vi "Excel Insert Header.vi"(7 "시트명":string="교정결과", 8 "error in":errorcluster caption="에러 입력(에러 없음)", 11 "report in":refnum<class "NI_report.lvclass">) -> (0 "error out":errorcluster, 3 "report out":refnum<class "NI_report.lvclass">, 4 "삭제에러":bool)   [LabVIEW 2020]
uses:
  <vilib>/Utility/NIReport.llb/NI_report.lvclass
  Controls/Cmd_Excel Insert Header.ctl
  <vilib>/Utility/error.llb/DialogType.ctl
  <vilib>/addons/_office/excel.llb/Excel Get Data ([str]).vi
  Variables/Global_Cal Info.vi
  <vilib>/Utility/error.llb/Error Cluster From Error Code.vi
  <vilib>/ErrorRing/Error Ring.xnode
  <vilib>/Utility/NIReport.llb/Excel/NI_Excel.lvclass
  <vilib>/addons/_office/NI_ReportGenerationToolkit.lvlib
panel:
  out "Header Lower":i32
  out "Header Upper":i32
  out "배열":string[][][](array[string])
  out "원소":string
  out "원소의 인덱스":i32
  out "Line":i32
  out "B_Tag Upper":i32
  out "B_Tag Lower":i32
  out "Header Column":i32
  out "?":T1
  out "Header Column":i32[](array[numeric])
  out "Header Row Count":i32[](array[numeric])
  out "Header Row":i32[](array[numeric])
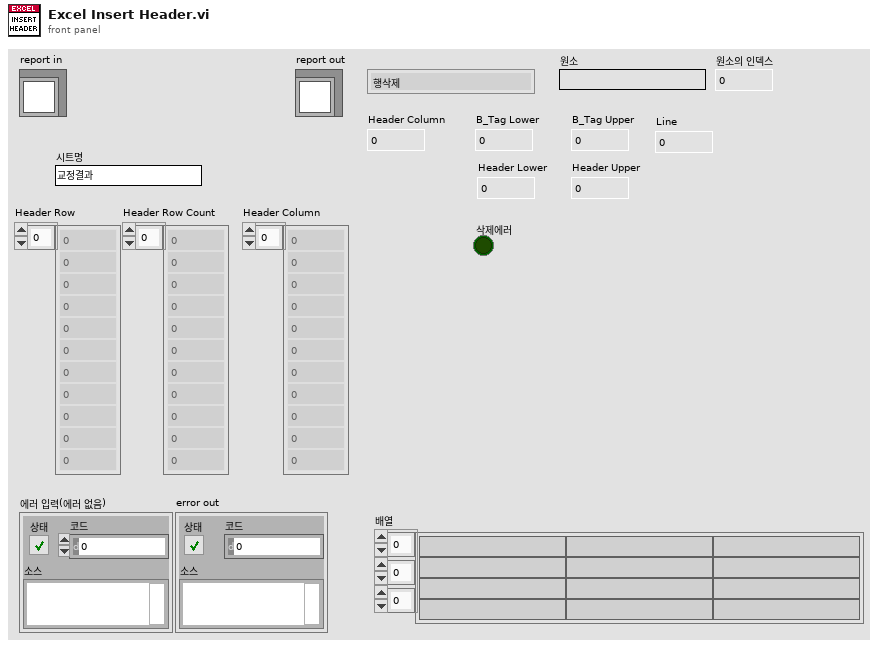
[diagram p1: front panel]
types:
  T1 = typedef "Cmd_Excel Insert Header.ctl" = enum16{"행삭제", "페이지 삭제", "B_Tag 읽기", "Header 읽기", "행 삽입", "Header 삽입", "Header 넘버링", "B_Tag 삽입", "오류 검사", "종료", "Error"}
  T2 = cluster{"position (excel)":cluster{"row":i32, "column":i32}, "name (excel)":string, "bookmark (word)":string}
  T3 = typedef "Clst_Cal Info Global.ctl" = cluster{"등록번호":string, "의뢰기관":string, "기기명":string, "제작회사":string, "형식":string, "기기번호":string, "소분류코드":string, "세부분류코드":string, "교정주기":string, "접수번호":string, "교정일자":string, "교정절차서 1":string, "교정절차서 2":string, "교정절차서 3":string, "접수확인자":string, "인증교정자":string, "기술책임자":string, "KOLAS 유무":string, "진행상태":string, "의뢰기관코드":string, "입고형태":string, "영문성적서?":bool, "합불판정?":bool, "부록?":bool, "절차서번호 1":string, "절차서번호 2":string, "절차서번호 3":string, "교정방식":string, "부서명":string}
  T4 = typedef "DialogType.ctl" = u16
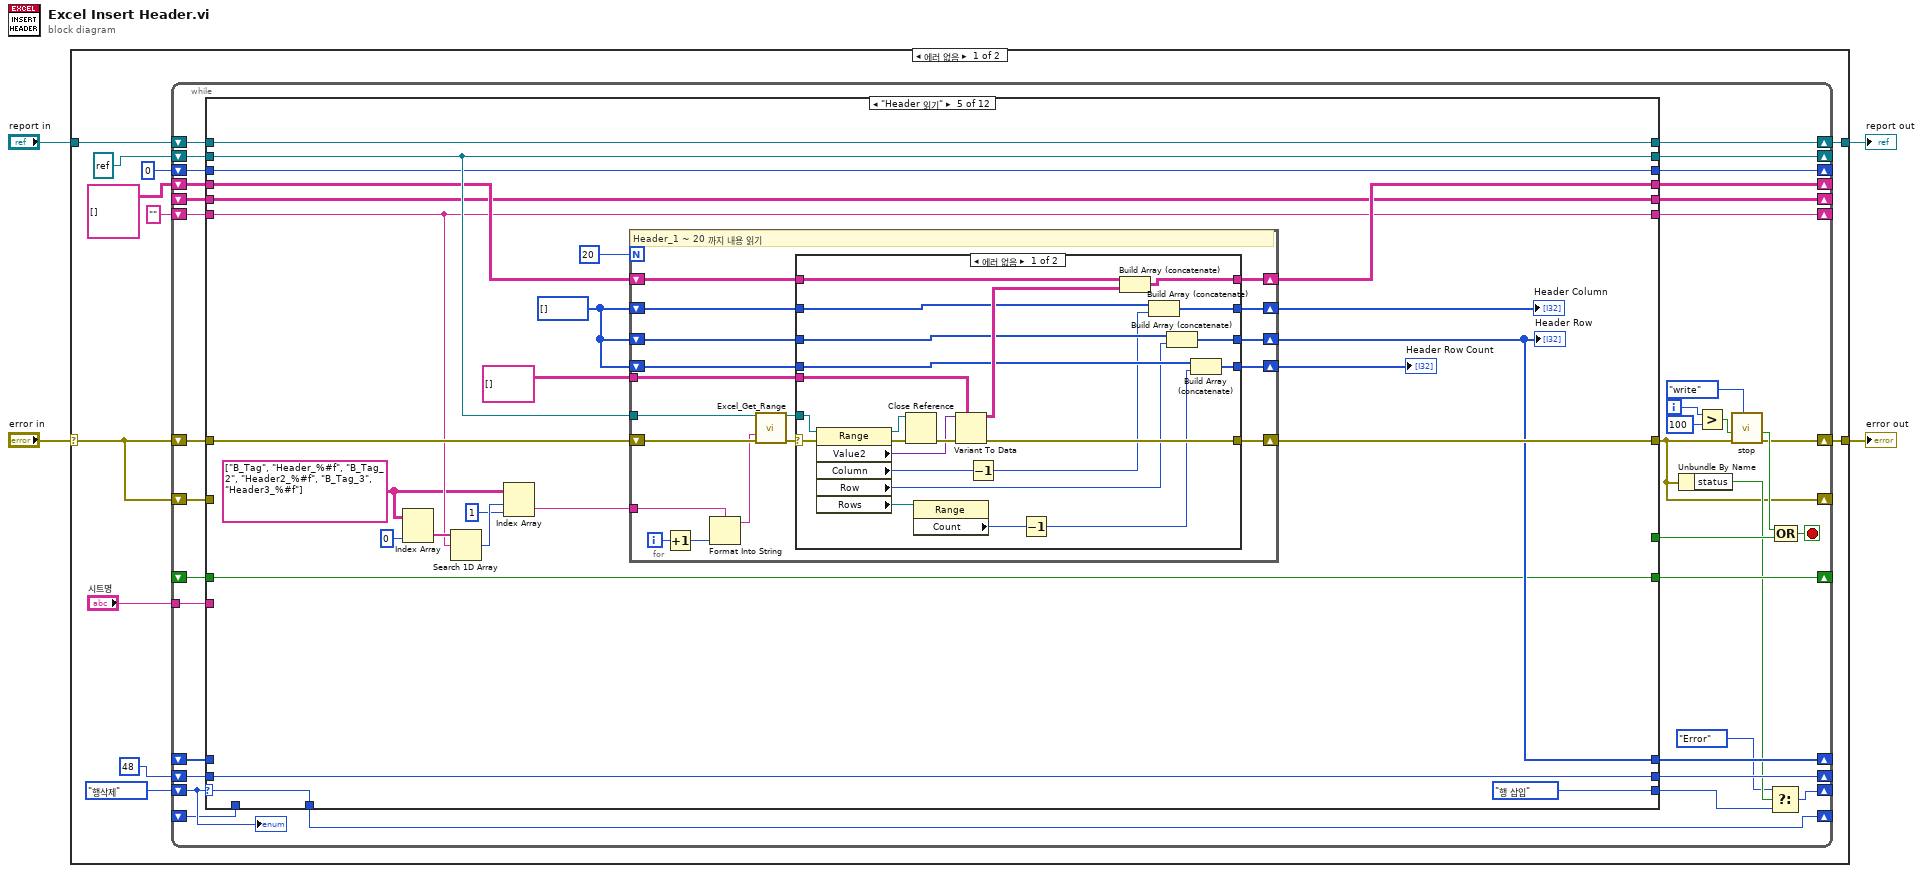
[diagram p0: block diagram]
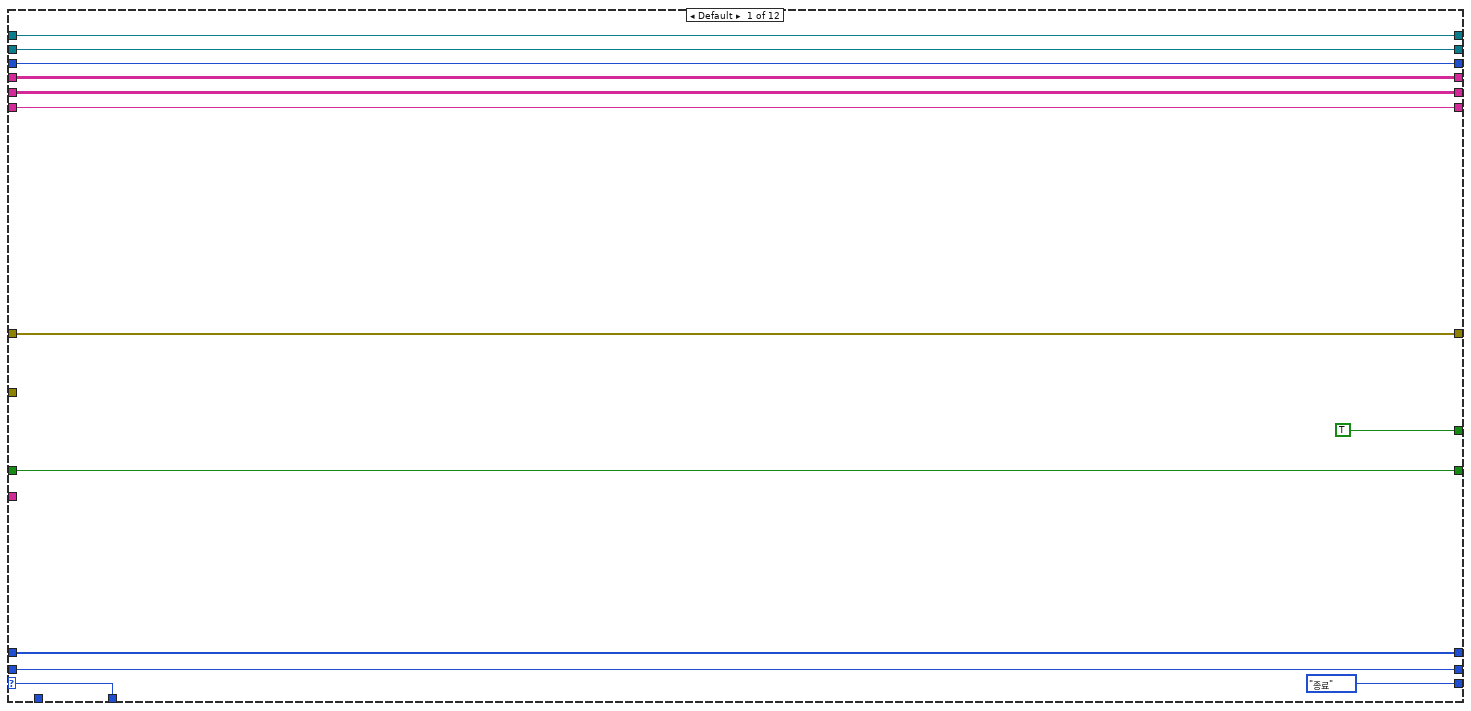
[diagram p2: hidden frame]
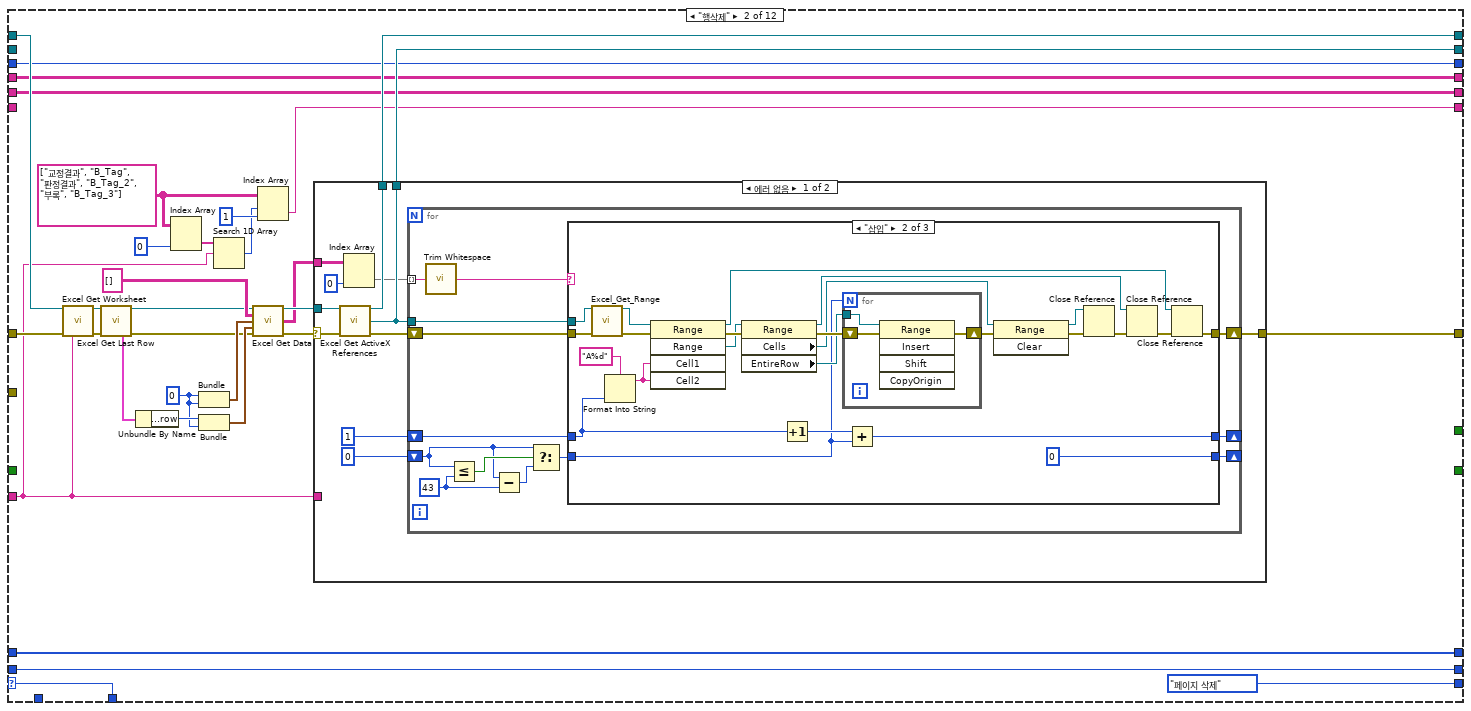
[diagram p3: hidden frame]
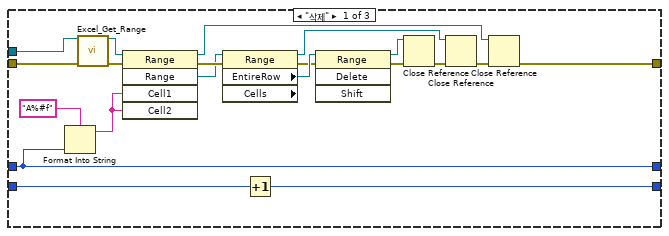
[diagram p4: hidden frame]
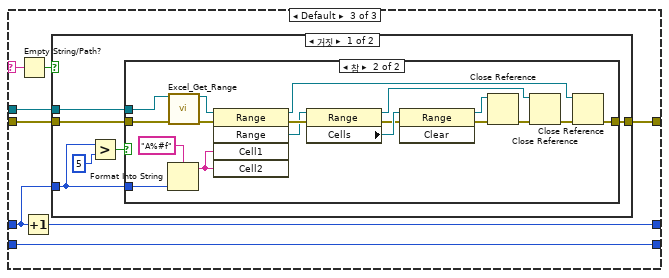
[diagram p5: hidden frame]
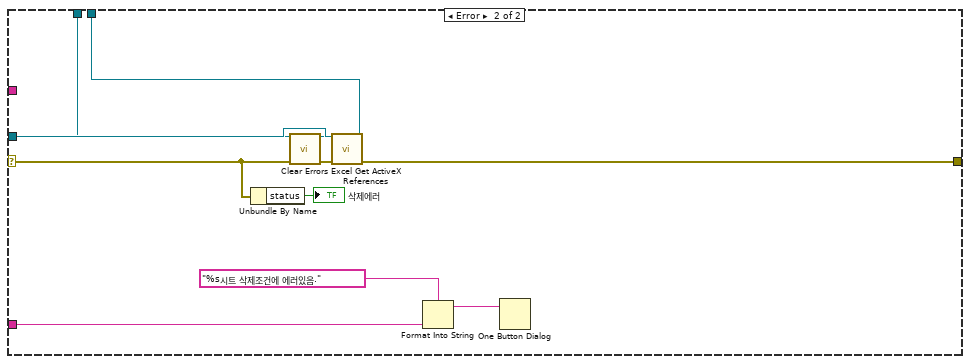
[diagram p8: hidden frame]
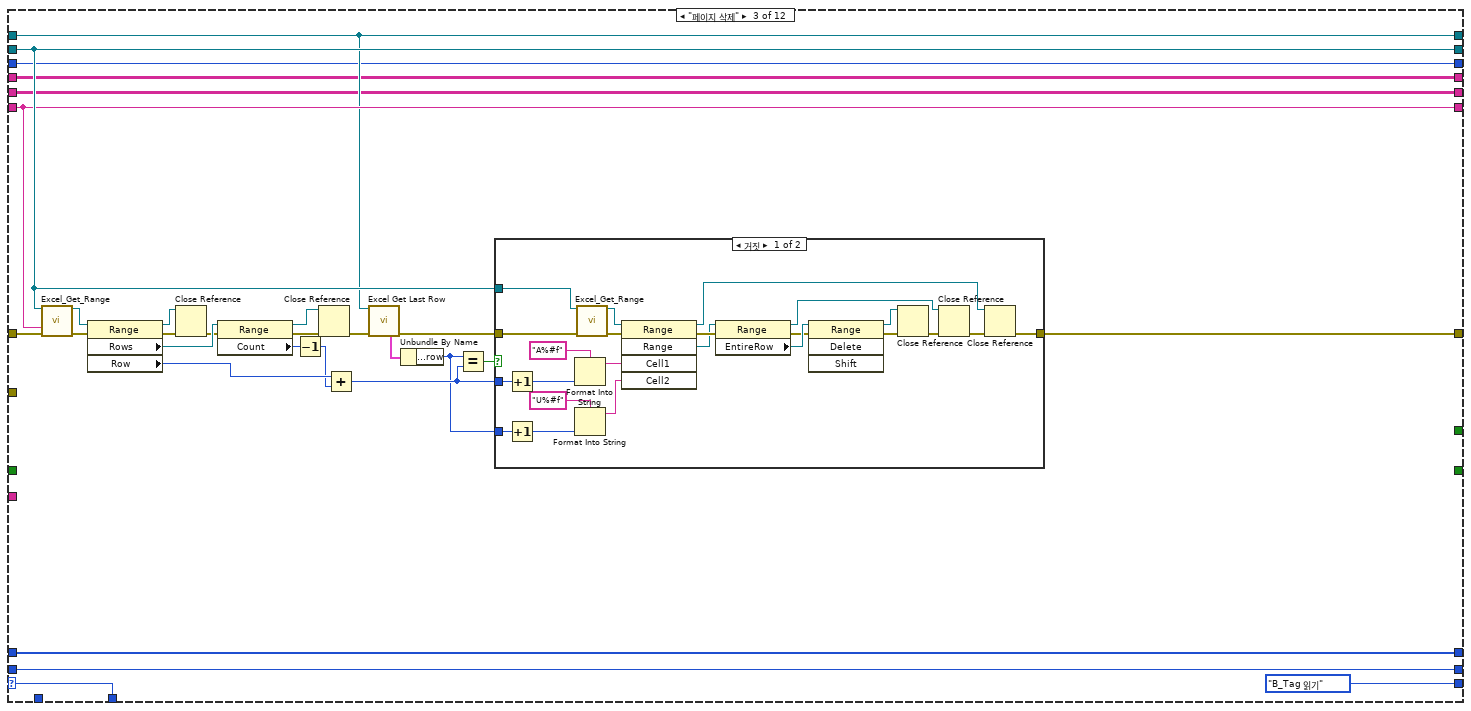
[diagram p9: hidden frame]
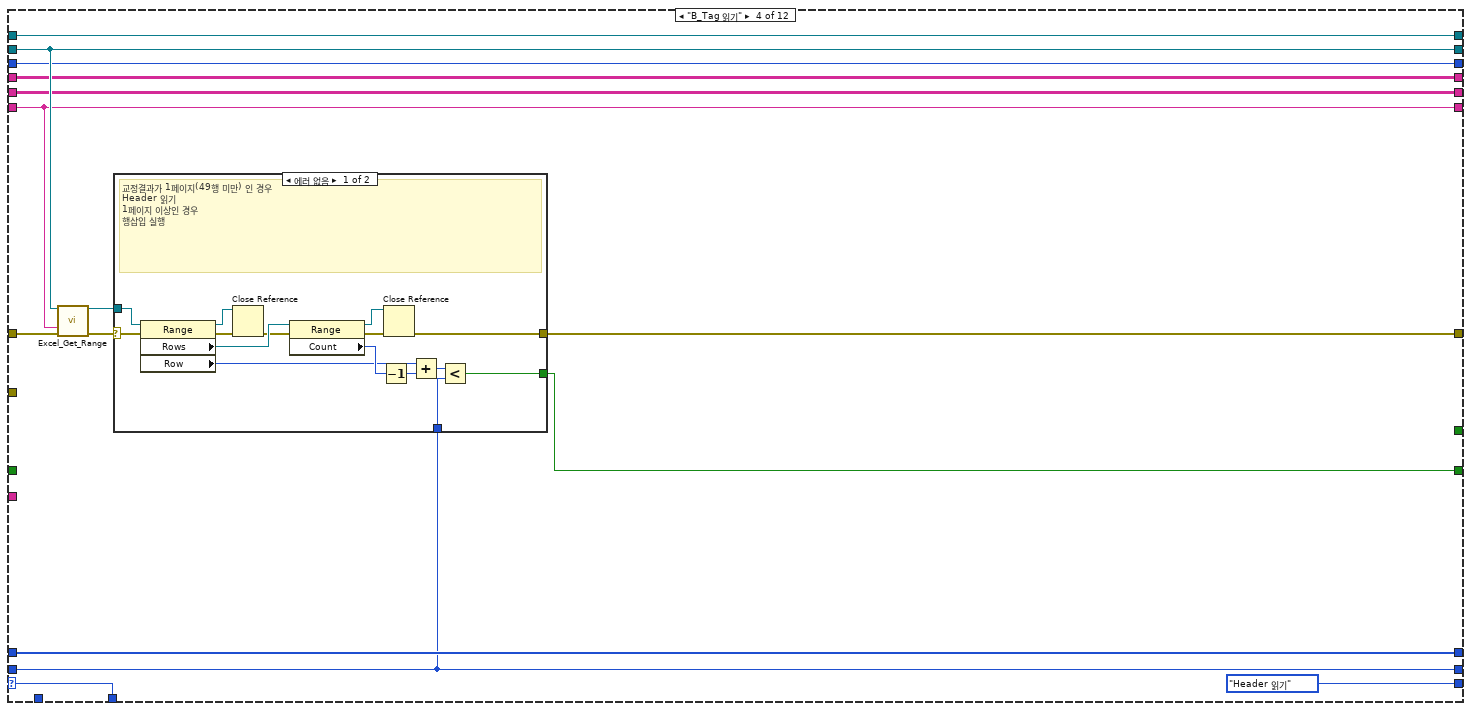
[diagram p11: hidden frame]
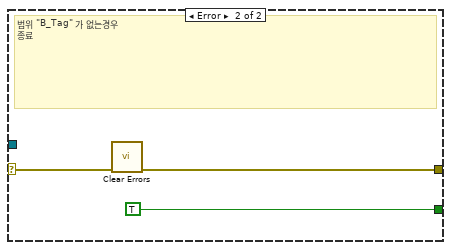
[diagram p12: hidden frame]
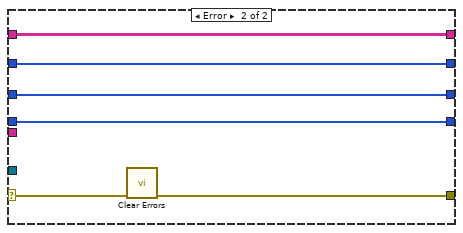
[diagram p13: hidden frame]
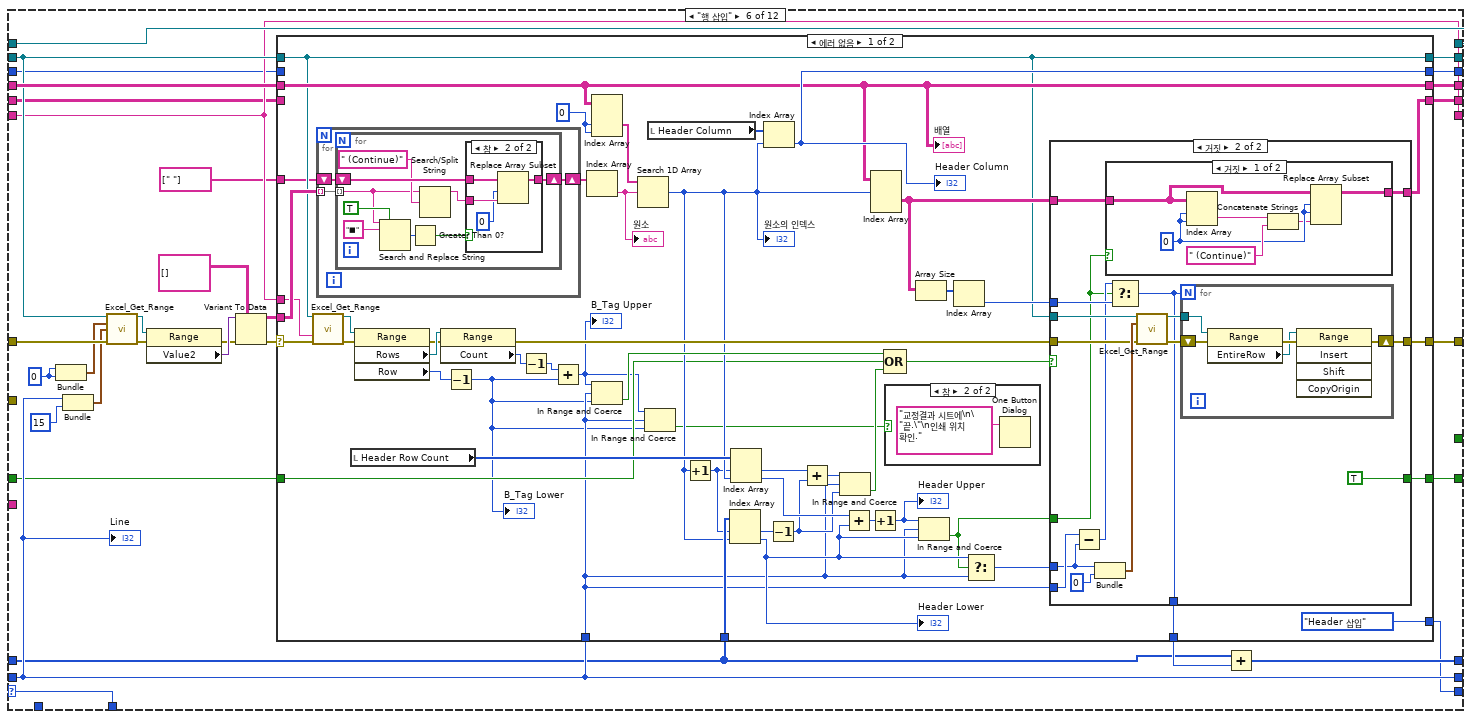
[diagram p14: hidden frame]
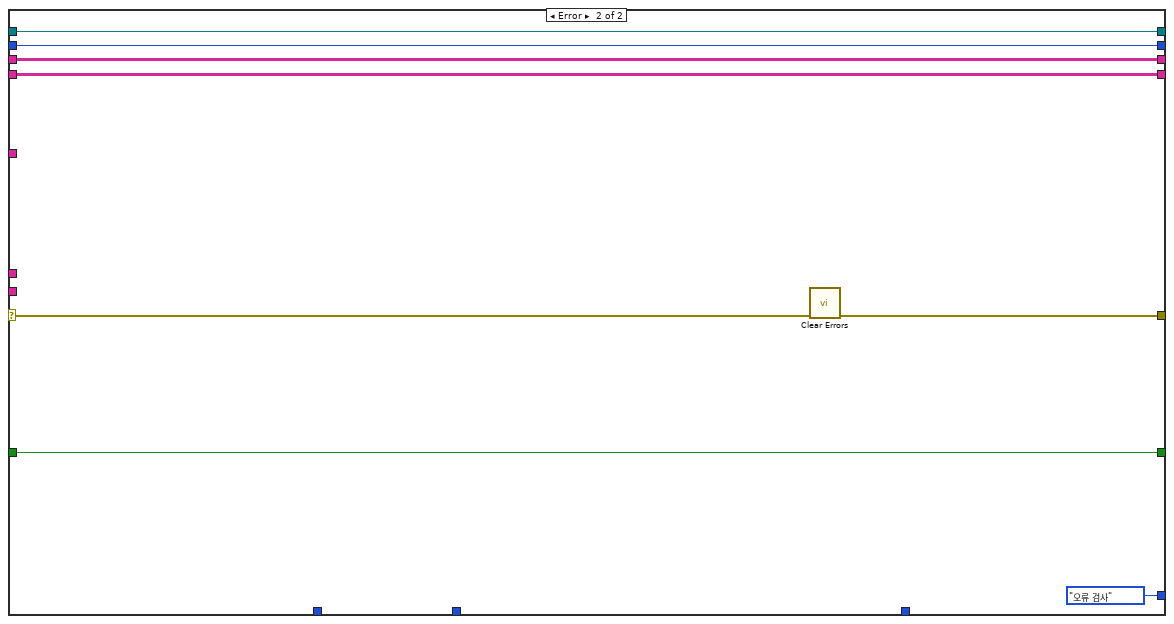
[diagram p19: hidden frame]
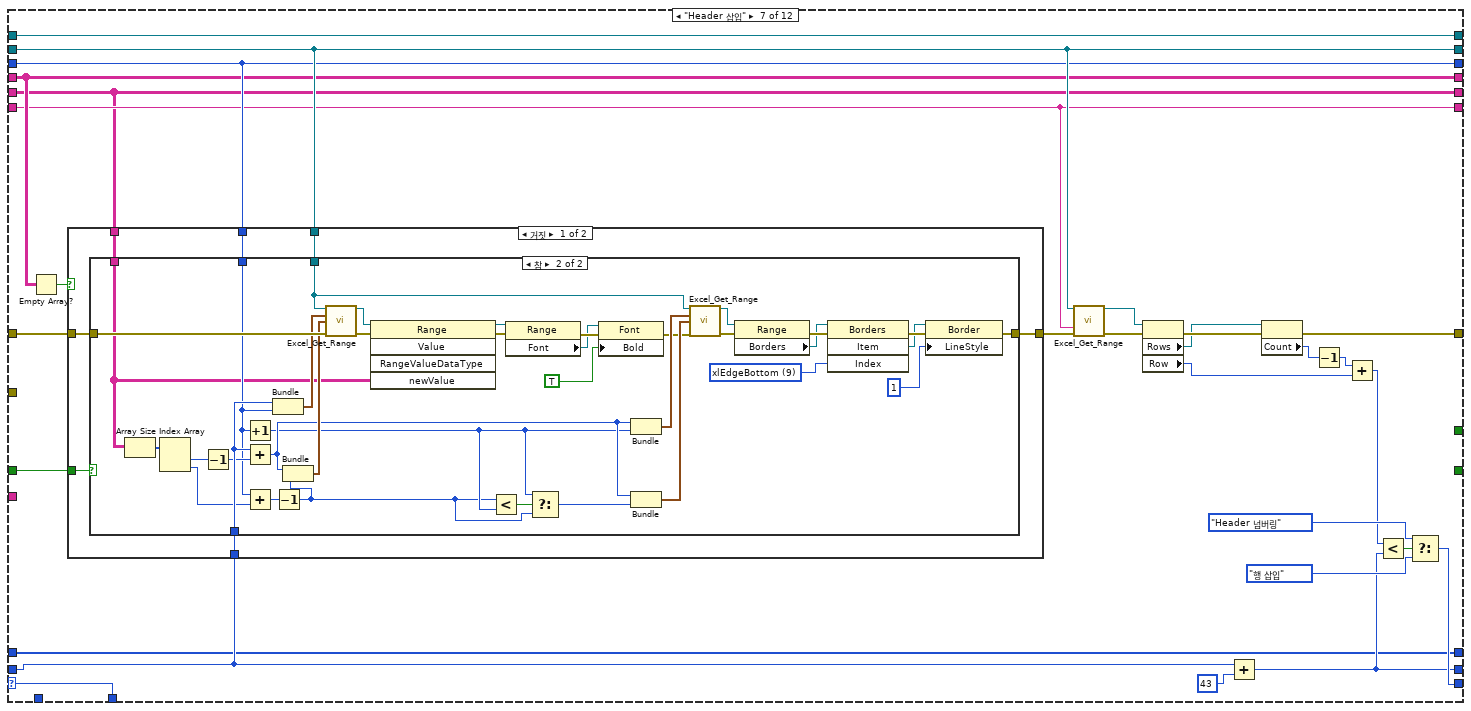
[diagram p20: hidden frame]
diagram:
  n1 = case shown="에러 없음" "error in" {
    selector: "error in" -> [w5 w784]
    tunnel: [w15 w784] -> w2
    tunnel: [w14 w783] -> w3
    tunnel: "report in" -> [w9 w783]
    frame No Error {
      n2 = while {
        shift-right: [w38] -> _
        shift-left: 48 -> [w29]
        shift-right: [w35] -> w15
        shift-left: w5 -> [w52]
        shift-right: [w22] -> _
        shift-left: Cmd_Excel_Insert_Header."행삭제" -> [w30]
        shift-right: [w51] -> w14
        shift-left: w9 -> [w50]
        shift-right: [w49] -> _
        shift-left: refnum<k7> refnum ("Excel._Worksheet") -> [w48]
        shift-right: [w47] -> _
        shift-left: string[][][] [] -> [w46]
        shift-right: [w37] -> _
        shift-left: 0 ("Column") -> [w36]
        shift-right: [w34] -> _
        shift-left: _ -> [w31]
        shift-right: [w32] -> _
        shift-left: _ -> [w33]
        shift-right: [w27] -> _
        shift-left: _ -> [w28]
        shift-right: [w25] -> _
        shift-left: "" -> [w26]
        tunnel: "시트명" -> [w24]
        shift-right: [w20] -> _
        shift-left: w5 -> [w19]
        shift-right: [w16] -> _
        shift-left: _ -> [w17]
        i -> [w42]
        stop <- w45 stop-if-true
        n3 = case shown="\"Header 읽기\"" w30 {
          selector: w30 -> [w53 w67 w213 w266 w299 w371 w508 w581 w663 w714 w748 w760]
          tunnel: [w55 w81 w223 w273 w317 w384 w517 w591 w702 w721 w753 w770] -> w38
          tunnel: w52 -> [w59 w86 w240 w276 w322 w401 w530 w600 w707 w727 w755 _]
          tunnel: [Cmd_Excel_Insert_Header."종료" Cmd_Excel_Insert_Header."페이지 삭제" Cmd_Excel_Insert_Header."B_Tag 읽기" Cmd_Excel_Insert_Header."Header 읽기" Cmd_Excel_Insert_Header."행 삽입" w378 w533 Cmd_Excel_Insert_Header."B_Tag 삽입" Cmd_Excel_Insert_Header."오류 검사" Cmd_Excel_Insert_Header."종료" Cmd_Excel_Insert_Header."종료" Cmd_Excel_Insert_Header."종료"] -> w18
          tunnel: [w65 w88 w222 w277 w320 w402 w532 w585 w706 w716 w759 w775] -> w51
          tunnel: w50 -> [w65 w84 w222 w277 w320 w402 w532 w599 w706 w725 w759 w775]
          tunnel: [w64 w87 w237 w275 w321 w374 w528 w596 w691 w724 w758 w774] -> w49
          tunnel: w48 -> [w64 _ w237 w275 w321 w386 w528 w596 w691 w724 w758 w774]
          tunnel: [w59 w80 w241 w278 w319 w392 w519 w586 w704 w726 w755 w764] -> w20
          tunnel: [w62 w75 w215 w268 w318 w379 w514 w592 w703 w722 w754 w771] -> w47
          tunnel: w46 -> [w62 w75 w215 w268 w311 w393 w514 w592 w703 w722 w754 w771]
          tunnel: [TRUE _ _ _ _ _ _ _ _ _ TRUE TRUE] -> w44
          tunnel: [w63 w76 w216 w269 w308 w388 w527 w587 w700 w718 w750 w767] -> w37
          tunnel: w36 -> [w63 w76 w216 w269 w308 w375 w527 w587 w700 w718 w750 w767]
          tunnel: [w58 _ _ w271 w307 w389 _ _ _ _ _ _] -> w34
          tunnel: w33 -> [w61 w74 w214 w267 w309 w373 w509 w588 w664 w717 w749 w766]
          tunnel: [w61 w74 w214 w267 w309 w387 w509 w588 w664 w717 w749 w766] -> w32
          tunnel: w31 -> [w58 _ _ _ w307 w377 w511 _ _ _ _ _]
          tunnel: w29 -> [w55 w81 w223 w273 w317 w384 w526 w591 w702 w721 w753 w770]
          tunnel: w28 -> [w56 w82 w239 w274 _ w381 w515 w590 w701 w720 w752 w769]
          tunnel: [w56 w82 w239 w274 w315 w382 w515 w590 w701 w720 w752 w769] -> w27
          tunnel: w26 -> [w60 _ w225 w270 w304 w376 w512 w589 w699 w719 w751 w768]
          tunnel: [w60 w68 w225 w270 w304 w376 w512 w589 w699 w719 w751 w768] -> w25
          tunnel: w24 -> [_ w66 _ _ _ _ _ _ _ w715 _ _]
          tunnel: w19 -> [_ _ _ _ _ _ _ _ _ _ _ _]
          tunnel: w17 -> [_ _ _ _ _ _ _ _ _ _ _ w761]
          tunnel: [w53 w67 w213 w266 w299 w371 w508 w581 w663 w714 w748 w760] -> w16
          frame Default {
          }
          frame "행삭제" {
            w71 = string[][] [["교정결과", "B_Tag"], ["판정결과", "B_Tag_2"], ["부록", "B_Tag_3"]]
            w78 = 0
            n4 = call <vilib>:"Excel Get Worksheet.vi"("report in"=w84, "error in (no error)"=w86, "name (\"\")"=w66) -> ("report out"=w83:refnum<class "NI_report.lvclass">, "error out"=w85:errorcluster)  [unwired: 11 in]
            n5 = call <vilib>:"Excel Get Last Row.vi"("report in"=w83, "error in (no error)"=w85) -> ("report out"=w91:refnum<class "NI_report.lvclass">, "MS Office parameters out"=w90:T2, "error out"=w92:errorcluster)  [unwired: 11 in]
            n6 = Unbundle By Name(w90) -> ("position (excel).row"=w95:i32)
            n7 = Index Array(array=w71, index (col)=0 ("비활성화된 인덱스 (열)")) -> (element=w72:string[])  [unwired: 1 in]
            n8 = Bundle(w78, w78) -> (w94:cluster{i32, i32})  [unwired: 1 in]
            n9 = Bundle("row"=w95, w78) -> (w96:cluster{"row":i32, i32})  [unwired: 1 in]
            n10 = Search 1D Array(1D array=w72, element=w66) -> (index of element=w69:i32)  [unwired: 1 in]
            n11 = call-poly <vilib>:"Excel Get Data.vi"("report in"=w91, "data type"=string[][] [], "start (-1, -1)"=w94, "end (-1, -1)"=w96, "error in (no error)"=w92) -> ("report out"=w97:refnum<class "NI_report.lvclass">, "data"=w89:string[][], "error out"=w79:errorcluster)  [unwired: 8 in]
            n12 = Index Array(array=w71, index (row)=w69, index (col)=1 ("비활성화된 인덱스 (열)")) -> (element=w68:string)
            n13 = case shown="에러 없음" w79 {
              selector: w79 -> [w101 w207]
              tunnel: w97 -> [w108 w212]
              tunnel: w89 -> [w100 _]
              tunnel: [w106 w211] -> w88
              tunnel: [w105 w210] -> w87
              tunnel: [w102 w209] -> w80
              tunnel: w66 -> [_ w205]
              frame No Error {
                n14 = call <vilib>:"Excel Get ActiveX References.vi"("report in"=w108, "error in (no error)"=w101) -> ("report out"=w106:refnum<class "NI_report.lvclass">, "Excel._Worksheet"=w105:refnum<k7>, "error out"=w107:errorcluster)  [unwired: 7 in, 4 out]
                n15 = Index Array(array=w100, index (col)=0 ("비활성화된 인덱스 (열)")) -> (element=w98:string[])  [unwired: 1 in]
                n16 = for {
                  tunnel: w98 -> [w115] mode=indexing
                  tunnel: w105 -> [w119]
                  shift-right: [w120] -> w102
                  shift-left: w107 -> [w121]
                  shift-right: [w117] -> _
                  shift-left: 1 -> [w118]
                  shift-right: [w116] -> _
                  shift-left: 0 -> [w111]
                  w110 = 43 ("y")
                  n17 = call <vilib>:"Trim Whitespace.vi"("string"=w115) -> ("trimmed string"=w114:string)  [unwired: 1 in]
                  n18 = Less Or Equal?(x=w111, y=w110) -> (x <= y?=w113:bool)
                  n19 = Subtract(x=w111, y=w110) -> (x-y=w109:i32)
                  n20 = Select(t=w111, s=w113, f=w109) -> (s? t:f=w112:i32)
                  n21 = case shown="\"삽입\"" w114 {
                    selector: w114 -> [_ _ w170]
                    tunnel: w121 -> [w140 w164 w175]
                    tunnel: [w128 w147 w174] -> w120
                    tunnel: w119 -> [w141 w165 w176]
                    tunnel: w118 -> [w126 w145 w171]
                    tunnel: [w126 w155 w172] -> w117
                    tunnel: w112 -> [w123 w142 w173]
                    tunnel: [w122 0 w173] -> w116
                    frame "삭제" {
                      n22 = Format Into String(format string="A%#f" ("문자열"), w126) -> (resulting string=w124:string)  [unwired: 2 in, 1 out]
                      n23 = call <vilib>:"Excel_Get_Range.vi"("Excel._Worksheet"=w141, "error in (no error)"=w140) -> ("Range"=w130:refnum<k7>, "error out"=w129:errorcluster)  [unwired: 12 in]
                      n24 = invoke class="Range" method="Range"(reference=w130, error in=w129, "Cell1"=w124, "Cell2"=w124) -> (reference out=w127:refnum<k7>, error out=w139:errorcluster, "Range"=w132:refnum<k7>)  [unwired: 1 in, 2 out]
                      n25 = property class="Range" props=["EntireRow", "Cells"](reference=w132, error in=w139) -> (reference out=w137:refnum<k7>, error out=w131:errorcluster, "EntireRow"=w133:refnum<k7>)  [unwired: 1 out]
                      n26 = Increment(x=w123) -> (x+1=w122:i32)
                      n27 = invoke class="Range" method="Delete"(reference=w133, error in=w131) -> (reference out=w136:refnum<k7>, error out=w138:errorcluster)  [unwired: 2 in, 2 out]
                      n28 = Close Reference(reference=w136, error in (no error)=w138) -> (error out=w135:errorcluster)
                      n29 = Close Reference(reference=w137, error in (no error)=w135) -> (error out=w134:errorcluster)
                      n30 = Close Reference(reference=w127, error in (no error)=w134) -> (error out=w128:errorcluster)
                    }
                    frame "삽입" {
                      n31 = call <vilib>:"Excel_Get_Range.vi"("Excel._Worksheet"=w165, "error in (no error)"=w164) -> ("Range"=w160:refnum<k7>, "error out"=w159:errorcluster)  [unwired: 12 in]
                      n32 = Format Into String(format string="A%d" ("문자열"), w145) -> (resulting string=w143:string)  [unwired: 2 in, 1 out]
                      n33 = invoke class="Range" method="Range"(reference=w160, error in=w159, "Cell1"=w143, "Cell2"=w143) -> (reference out=w148:refnum<k7>, error out=w163:errorcluster, "Range"=w162:refnum<k7>)  [unwired: 1 in, 2 out]
                      n34 = property class="Range"(reference=w162, error in=w163) -> (reference out=w150:refnum<k7>, error out=w161:errorcluster, "Cells"=w158:refnum<k7>, "EntireRow"=w146:refnum<k7>)
                      n35 = Increment(x=w145) -> (x+1=w154:i32)
                      n36 = for {
                        N: w142 -> [_]
                        tunnel: w146 -> [w168]
                        shift-right: [w166] -> w157
                        shift-left: w161 -> [w167]
                        n37 = invoke class="Range" method="Insert"(reference=w168, error in=w167) -> (error out=w166:errorcluster)  [unwired: 3 in, 4 out]
                      }
                      n38 = Add(x=w154, y=w142) -> (x+y=w155:i32)
                      n39 = invoke class="Range" method="Clear"(reference=w158, error in=w157) -> (reference out=w153:refnum<k7>, error out=w152:errorcluster)  [unwired: 1 in, 1 out]
                      n40 = Close Reference(reference=w153, error in (no error)=w152) -> (error out=w151:errorcluster)
                      n41 = Close Reference(reference=w150, error in (no error)=w151) -> (error out=w149:errorcluster)
                      n42 = Close Reference(reference=w148, error in (no error)=w149) -> (error out=w147:errorcluster)
                    }
                    frame Default {
                      n43 = Empty String/Path?(string/path=w170) -> (empty?=w169:bool)
                      n44 = Increment(x=w171) -> (x+1=w172:i32)
                      n45 = case shown="거짓" w169 {
                        tunnel: w176 -> [w182 _]
                        tunnel: w175 -> [w181 w202]
                        tunnel: [w180 w202] -> w174
                        tunnel: w171 -> [w179 _]
                        frame False {
                          n46 = Greater?(x=w179, y=5) -> (0:w177:bool)
                          n47 = case shown="참" w177 {
                            tunnel: w182 -> [_ w201]
                            tunnel: w181 -> [w183 w200]
                            tunnel: [w183 w188] -> w180
                            tunnel: w179 -> [_ w184]
                            frame False {
                            }
                            frame True {
                              n48 = Format Into String(format string="A%#f" ("문자열"), w184) -> (resulting string=w185:string)  [unwired: 2 in, 1 out]
                              n49 = call <vilib>:"Excel_Get_Range.vi"("Excel._Worksheet"=w201, "error in (no error)"=w200) -> ("Range"=w190:refnum<k7>, "error out"=w189:errorcluster)  [unwired: 12 in]
                              n50 = invoke class="Range" method="Range"(reference=w190, error in=w189, "Cell1"=w185, "Cell2"=w185) -> (reference out=w187:refnum<k7>, error out=w199:errorcluster, "Range"=w192:refnum<k7>)  [unwired: 1 in, 2 out]
                              n51 = property class="Range"(reference=w192, error in=w199) -> (reference out=w197:refnum<k7>, error out=w191:errorcluster, "Cells"=w193:refnum<k7>)
                              n52 = invoke class="Range" method="Clear"(reference=w193, error in=w191) -> (reference out=w196:refnum<k7>, error out=w198:errorcluster)  [unwired: 1 in, 1 out]
                              n53 = Close Reference(reference=w196, error in (no error)=w198) -> (error out=w195:errorcluster)
                              n54 = Close Reference(reference=w197, error in (no error)=w195) -> (error out=w194:errorcluster)
                              n55 = Close Reference(reference=w187, error in (no error)=w194) -> (error out=w188:errorcluster)
                            }
                          }
                        }
                        frame True {
                        }
                      }
                    }
                  }
                }
              }
              frame Error {
                n56 = Unbundle By Name(w207) -> ("status"=→"삭제에러":bool)
                n57 = call <vilib>:"Clear Errors.vi"("error in (no error)"=w207) -> ("error out"=w208:errorcluster)  [unwired: 5 in, 1 out]
                n58 = call <vilib>:"Excel Get ActiveX References.vi"("report in"=w212, "error in (no error)"=w208) -> ("report out"=w211:refnum<class "NI_report.lvclass">, "Excel._Worksheet"=w210:refnum<k7>, "error out"=w209:errorcluster)  [unwired: 7 in, 4 out]
                n59 = Format Into String(format string="%s시트 삭제조건에 에러있음." ("메시지"), w205) -> (resulting string=w203:string)  [unwired: 2 in, 1 out]
                n60 = One Button Dialog(message=w203) -> ()  [unwired: 1 in, 1 out]
              }
            }
          }
          frame "페이지 삭제" {
            n61 = call <vilib>:"Excel_Get_Range.vi"("Excel._Worksheet"=w237, "name"=w225, "error in (no error)"=w240) -> ("Range"=w226:refnum<k7>, "error out"=w228:errorcluster)  [unwired: 11 in]
            n62 = property class="Range"(reference=w226, error in=w228) -> (reference out=w235:refnum<k7>, error out=w236:errorcluster, "Rows"=w234:refnum<k7>, "Row"=w231:i32)
            n63 = Close Reference(reference=w235, error in (no error)=w236) -> (error out=w232:errorcluster)
            n64 = property class="Range"(reference=w234, error in=w232) -> (reference out=w229:refnum<k7>, error out=w230:errorcluster, "Count"=w233:i32)
            n65 = Decrement(x=w233) -> (x-1=w224:i32)
            n66 = Close Reference(reference=w229, error in (no error)=w230) -> (error out=w227:errorcluster)
            n67 = Add(x=w231, y=w224) -> (x+y=w219:i32)
            n68 = call <vilib>:"Excel Get Last Row.vi"("report in"=w222, "error in (no error)"=w227) -> ("MS Office parameters out"=w221:T2, "error out"=w220:errorcluster)  [unwired: 11 in, 1 out]
            n69 = Unbundle By Name(w221) -> ("position (excel).row"=w218:i32)
            n70 = Equal?(x=w218, y=w219) -> (x = y?=w217:bool)
            n71 = case shown="거짓" w217 {
              tunnel: [w242 w265] -> w241
              tunnel: w237 -> [w264 _]
              tunnel: w220 -> [w253 w265]
              tunnel: w219 -> [w252 _]
              tunnel: w218 -> [w251 _]
              frame False {
                n72 = Increment(x=w252) -> (x+1=w250:i32)
                n73 = Increment(x=w251) -> (x+1=w249:i32)
                n74 = Format Into String(format string="A%#f" ("문자열"), w250) -> (resulting string=w256:string)  [unwired: 2 in, 1 out]
                n75 = Format Into String(format string="U%#f" ("문자열"), w249) -> (resulting string=w254:string)  [unwired: 2 in, 1 out]
                n76 = call <vilib>:"Excel_Get_Range.vi"("Excel._Worksheet"=w264, "error in (no error)"=w253) -> ("Range"=w259:refnum<k7>, "error out"=w258:errorcluster)  [unwired: 12 in]
                n77 = invoke class="Range" method="Range"(reference=w259, error in=w258, "Cell1"=w256, "Cell2"=w254) -> (reference out=w243:refnum<k7>, error out=w263:errorcluster, "Range"=w261:refnum<k7>)  [unwired: 1 in, 2 out]
                n78 = property class="Range"(reference=w261, error in=w263) -> (reference out=w245:refnum<k7>, error out=w260:errorcluster, "EntireRow"=w262:refnum<k7>)
                n79 = invoke class="Range" method="Delete"(reference=w262, error in=w260) -> (reference out=w247:refnum<k7>, error out=w248:errorcluster)  [unwired: 2 in, 2 out]
                n80 = Close Reference(reference=w247, error in (no error)=w248) -> (error out=w246:errorcluster)
                n81 = Close Reference(reference=w245, error in (no error)=w246) -> (error out=w244:errorcluster)
                n82 = Close Reference(reference=w243, error in (no error)=w244) -> (error out=w242:errorcluster)
              }
              frame True {
              }
            }
          }
          frame "B_Tag 읽기" {
            n83 = call <vilib>:"Excel_Get_Range.vi"("Excel._Worksheet"=w275, "name"=w270, "error in (no error)"=w276) -> ("Range"=w279:refnum<k7>, "error out"=w280:errorcluster)  [unwired: 11 in]
            n84 = case shown="에러 없음" w280 {
              selector: w280 -> [w292 w296]
              tunnel: [w282 TRUE] -> w271
              tunnel: [w284 w297] -> w278
              tunnel: w279 -> [w295 _]
              tunnel: w273 -> [w291 _]
              frame No Error {
                # "교정결과가 1페이지(49행 미만) 인 경우\nHeader 읽기\n1페이지 이상인 경우 \n행삽입 실행"
                n85 = property class="Range"(reference=w295, error in=w292) -> (reference out=w293:refnum<k7>, error out=w294:errorcluster, "Rows"=w290:refnum<k7>, "Row"=w286:i32)
                n86 = Close Reference(reference=w293, error in (no error)=w294) -> (error out=w287:errorcluster)
                n87 = property class="Range"(reference=w290, error in=w287) -> (reference out=w283:refnum<k7>, error out=w285:errorcluster, "Count"=w289:i32)
                n88 = Decrement(x=w289) -> (x-1=w281:i32)
                n89 = Close Reference(reference=w283, error in (no error)=w285) -> (error out=w284:errorcluster)
                n90 = Add(x=w286, y=w281) -> (x+y=w288:i32)
                n91 = Less?(x=w288, y=w291) -> (x < y?=w282:bool)
              }
              frame Error {
                # "범위 \"B_Tag\" 가 없는경우\n종료"
                n92 = call <vilib>:"Clear Errors.vi"("error in (no error)"=w296) -> ("error out"=w297:errorcluster)  [unwired: 5 in, 1 out]
              }
            }
          }
          frame "Header 읽기" {
            w303 = string[][] [["B_Tag", "Header_%#f"], ["B_Tag_2", "Header2_%#f"], ["B_Tag_3", "Header3_%#f"]]
            w313 = i32[] []
            n93 = Index Array(array=w303, index (col)=0 ("비활성화된 인덱스 (열)")) -> (element=w305:string[])  [unwired: 1 in]
            n94 = Search 1D Array(1D array=w305, element=w304) -> (index of element=w302:i32)  [unwired: 1 in]
            n95 = Index Array(array=w303, index (row)=w302, index (col)=1 ("비활성화된 인덱스 (열)")) -> (element=w300:string)
            n96 = for {
              N: 20 -> [_]
              shift-right: [w337] -> w319
              shift-left: w322 -> [w341]
              tunnel: w321 -> [w339]
              shift-right: [w336] -> w318
              shift-left: w311 -> [w335]
              shift-right: [w331] -> w316
              shift-left: w313 -> [w330]
              shift-right: [w328] -> w315
              shift-left: w313 -> [w329]
              shift-right: [w326] -> w314
              shift-left: w313 -> [w327]
              tunnel: w300 -> [w325]
              tunnel: string[][] [] -> [w324]
              i -> [w340]
              # "Header_1 ~ 20 까지 내용 읽기"
              n97 = Increment(x=w340) -> (x+1=w332:i32)
              n98 = Format Into String(format string=w325, w332) -> (resulting string=w334:string)  [unwired: 2 in, 1 out]
              n99 = call <vilib>:"Excel_Get_Range.vi"("Excel._Worksheet"=w339, "name"=w334, "error in (no error)"=w341) -> ("Range"=w338:refnum<k7>, "error out"=w333:errorcluster)  [unwired: 11 in]
              n100 = case shown="에러 없음" w333 {
                selector: w333 -> [w356 w370]
                tunnel: w338 -> [w364 _]
                tunnel: [w359 w369] -> w337
                tunnel: [w358 w368] -> w336
                tunnel: w335 -> [w357 w368]
                tunnel: [w352 w367] -> w331
                tunnel: w330 -> [w351 w367]
                tunnel: w329 -> [w350 w366]
                tunnel: [w349 w366] -> w328
                tunnel: w327 -> [w348 w365]
                tunnel: [w347 w365] -> w326
                tunnel: w324 -> [w345 _]
                frame No Error {
                  n101 = property class="Range"(reference=w364, error in=w356) -> (reference out=w363:refnum<k7>, error out=w362:errorcluster, "Value2"=w360:variant, "Column"=w353:i32, "Row"=w344:i32, "Rows"=w354:refnum<k7>)
                  n102 = Close Reference(reference=w363, error in (no error)=w362) -> (error out=w361:errorcluster)
                  n103 = property class="Range"(reference=w354) -> ("Count"=w343:i32)  [unwired: 1 in, 2 out]
                  n104 = Variant To Data(error in=w361, type=w345, Variant=w360) -> (data=w355:string[][], error out=w359:errorcluster)
                  n105 = Decrement(x=w353) -> (x-1=w346:i32)
                  n106 = Decrement(x=w343) -> (x-1=w342:i32)
                  n107 = Build Array (concatenate)(w357, w355) -> (w358:string[][][])
                  n108 = Build Array (concatenate)(w351, w346) -> (w352:i32[])
                  n109 = Build Array (concatenate)(w350, w344) -> (w349:i32[])
                  n110 = Build Array (concatenate)(w348, w342) -> (w347:i32[])
                }
                frame Error {
                  n111 = call <vilib>:"Clear Errors.vi"("error in (no error)"=w370) -> ("error out"=w369:errorcluster)  [unwired: 5 in, 1 out]
                }
              }
            }
            "Header Row" <- w315
            "Header Row Count" <- w314
            "Header Column" <- w316
          }
          frame "행 삽입" {
            w391 = 0
            n112 = Bundle(w391, w391) -> (w400:cluster{i32, i32})  [unwired: 1 in]
            n113 = Bundle(w384, "column"=15) -> (w399:cluster{i32, "column":i32})  [unwired: 1 in]
            n114 = call <vilib>:"Excel_Get_Range.vi"("Excel._Worksheet"=w386, "start"=w400, "end"=w399, "error in (no error)"=w401) -> ("Range"=w397:refnum<k7>, "error out"=w398:errorcluster)  [unwired: 10 in]
            n115 = property class="Range"(reference=w397, error in=w398) -> (error out=w385:errorcluster, "Value2"=w396:variant)  [unwired: 1 out]
            n116 = Variant To Data(error in=w385, type=string[][] [], Variant=w396) -> (data=w395:string[][], error out=w380:errorcluster)
            n117 = case shown="에러 없음" w380 {
              selector: w380 -> [w425 w507]
              tunnel: w395 -> [w452 _]
              tunnel: w393 -> [w424 w502]
              tunnel: [w447 w506] -> w392
              tunnel: [w443 w500] -> w389
              tunnel: [w441 w504] -> w388
              tunnel: [w439 w501] -> w387
              tunnel: w386 -> [w404 w503]
              tunnel: w384 -> [w407 _]
              tunnel: [w427 _] -> w383
              tunnel: w381 -> [w426 _]
              tunnel: [w424 w502] -> w379
              tunnel: [Cmd_Excel_Insert_Header."Header 삽입" Cmd_Excel_Insert_Header."오류 검사"] -> w378
              tunnel: w377 -> [w415 w500]
              tunnel: w376 -> [w421 _]
              tunnel: w375 -> [_ w504]
              tunnel: [w404 w503] -> w374
              tunnel: w373 -> [_ w501]
              tunnel: string[] [" "] -> [w403 _]
              frame No Error {
                w451 = 0 ("인덱스 (페이지)")
                n118 = call <vilib>:"Excel_Get_Range.vi"("Excel._Worksheet"=w404, "name"=w421, "error in (no error)"=w425) -> ("Range"=w438:refnum<k7>, "error out"=w437:errorcluster)  [unwired: 11 in]
                n119 = for {
                  tunnel: w452 -> [w485] mode=indexing
                  shift-right: [w483] -> w449
                  shift-left: w403 -> [w484]
                  n120 = for {
                    tunnel: w485 -> [w487] mode=indexing
                    shift-right: [w490] -> w483
                    shift-left: w484 -> [w491]
                    n121 = Search and Replace String(replace all?=TRUE ("모두 대체? (거짓)"), input string=w487, search string="■" ("검색 문자열")) -> (number of replacements=w493:i32)  [unwired: 5 in, 3 out]
                    n122 = Greater Than 0?(x=w493) -> (x > 0?=w492:bool)
                    n123 = Search/Split String(string=w487, search string/char (-)=" (Continue)" ("문자열")) -> (substring before match=w486:string)  [unwired: 1 in, 2 out]
                    n124 = case shown="참" w492 {
                      tunnel: w491 -> [w495 w499]
                      tunnel: [w495 w498] -> w490
                      tunnel: w486 -> [_ w497]
                      frame False {
                      }
                      frame True {
                        n125 = Replace Array Subset(array=w499, new element=w497, index=0 ("인덱스")) -> (w498:string[])
                      }
                    }
                  }
                }
                n126 = local read "Header Row Count"() -> (w446:i32[])
                n127 = property class="Range"(reference=w438, error in=w437) -> (error out=w435:errorcluster, "Rows"=w436:refnum<k7>, "Row"=w433:i32)  [unwired: 1 out]
                n128 = property class="Range"(reference=w436, error in=w435) -> (error out=w434:errorcluster, "Count"=w432:i32)  [unwired: 1 out]
                n129 = Decrement(x=w433) -> (x-1=w405:i32)
                "B_Tag Lower" <- w405
                n130 = Decrement(x=w432) -> (x-1=w417:i32)
                n131 = Add(x=w417, y=w405) -> (x+y=w406:i32)
                "B_Tag Upper" <- w406
                n132 = Index Array(array=w449) -> (element=w448:string)  [unwired: 1 in]
                "원소" <- w448
                n133 = Index Array(array=w424, index (dim 1)=w451, index (dim 2)=w451) -> (element=w450:string[])  [unwired: 1 in]
                n134 = In Range and Coerce(upper limit=w406, x=w407, lower limit=w405) -> (In Range?=w422:bool)  [unwired: 1 out]
                n135 = Search 1D Array(1D array=w450, element=w448) -> (index of element=w420:i32)  [unwired: 1 in]
                "원소의 인덱스" <- w420
                n136 = In Range and Coerce(upper limit=w406, x=w407, lower limit=w405) -> (In Range?=w408:bool)  [unwired: 1 out]
                n137 = local read "Header Column"() -> (w442:i32[])
                n138 = Increment(x=w420) -> (x+1=w413:i32)
                n139 = Index Array(array=w426, index #1=w413, index #2=w420) -> (element #1=w412:i32, element #2=w430:i32)
                "Header Lower" <- w430
                n140 = Index Array(array=w446, index #1=w413, index #2=w420) -> (element #1=w414:i32, element #2=w431:i32)
                n141 = Index Array(array=w442, index=w420) -> (element=w441:i32)
                "Header Column" <- w441
                n142 = Decrement(x=w412) -> (x-1=w411:i32)
                n143 = Add(x=w414, y=w411) -> (x+y=w418:i32)
                n144 = In Range and Coerce(upper limit=w418, x=w407, lower limit=w411) -> (In Range?=w416:bool)  [unwired: 1 out]
                n145 = Add(x=w431, y=w430) -> (x+y=w428:i32)
                n146 = Increment(x=w428) -> (x+1=w409:i32)
                "Header Upper" <- w409
                n147 = Index Array(array=w424, index (dim 0)=w420) -> (element=w440:string[][])  [unwired: 2 in]
                n148 = Compound Arithmetic op=OR(w422, w415, w416) -> (w419:bool)
                n149 = case shown="참" w408 {
                  frame False {
                  }
                  frame True {
                    n150 = One Button Dialog(message="교정결과 시트에\n\"끝.\"\n인쇄 위치 확인." ("메시지")) -> ()  [unwired: 1 in, 1 out]
                  }
                }
                n151 = Array Size(array=w440) -> (size(s)=w445:i32[])
                n152 = In Range and Coerce(upper limit=w409, x=w407, lower limit=w430) -> (In Range?=w410:bool)  [unwired: 1 out]
                n153 = Index Array(array=w445) -> (element=w444:i32)  [unwired: 1 in]
                n154 = Select(t=w430, s=w410, f=w407) -> (s? t:f=w429:i32)
                n155 = case shown="거짓" w419 {
                  tunnel: w404 -> [_ w467]
                  tunnel: w434 -> [w454 w466]
                  tunnel: w429 -> [_ w464]
                  tunnel: [w454 w458] -> w447
                  tunnel: w444 -> [_ w463]
                  tunnel: w407 -> [_ w465]
                  tunnel: w410 -> [_ w456]
                  tunnel: [_ TRUE] -> w443
                  tunnel: w440 -> [_ w461]
                  tunnel: [_ w460] -> w439
                  tunnel: [_ w457] -> w427
                  frame True {
                  }
                  frame False {
                    n156 = Subtract(x=w465, y=w464) -> (x-y=w462:i32)
                    n157 = Bundle(w464, "인덱스 (페이지)"=0) -> (w468:cluster{i32, "인덱스 (페이지)":i32})  [unwired: 1 in]
                    n158 = case shown="거짓" w456 {
                      tunnel: w461 -> [w474 w477]
                      tunnel: [w471 w477] -> w460
                      frame False {
                        w473 = 0 ("인덱스 (행)")
                        n159 = Index Array(array=w474, index (row)=w473, index (col)=w473) -> (element=w476:string)
                        n160 = Concatenate Strings(w476, " (Continue)" ("문자열")) -> (w472:string)
                        n161 = Replace Array Subset(array=w474, new element=w472, index (row)=w473, index (col)=w473) -> (w471:string[][])
                      }
                      frame True {
                      }
                    }
                    n162 = Select(t=w462, s=w456, f=w463) -> (s? t:f=w457:i32)
                    n163 = call <vilib>:"Excel_Get_Range.vi"("Excel._Worksheet"=w467, "start"=w468, "error in (no error)"=w466) -> ("Range"=w469:refnum<k7>, "error out"=w470:errorcluster)  [unwired: 11 in]
                    n164 = for {
                      N: w457 -> [_]
                      tunnel: w469 -> [w479]
                      shift-right: [w478] -> w458
                      shift-left: w470 -> [w482]
                      n165 = property class="Range"(reference=w479, error in=w482) -> (error out=w481:errorcluster, "EntireRow"=w480:refnum<k7>)  [unwired: 1 out]
                      n166 = invoke class="Range" method="Insert"(reference=w480, error in=w481) -> (error out=w478:errorcluster)  [unwired: 3 in, 4 out]
                    }
                  }
                }
                "배열" <- w424
              }
              frame Error {
                n167 = call <vilib>:"Clear Errors.vi"("error in (no error)"=w507) -> ("error out"=w506:errorcluster)  [unwired: 5 in, 1 out]
              }
            }
            n168 = Add(x=w381, y=w383) -> (x+y=w382:i32[])
            "Line" <- w384
          }
          frame "Header 삽입" {
            n169 = Empty Array?(array=w514) -> (empty?=w513:bool)
            n170 = case shown="거짓" w513 {
              tunnel: w530 -> [w542 w580]
              tunnel: [w541 w580] -> w529
              tunnel: w528 -> [w540 _]
              tunnel: w509 -> [w539 _]
              tunnel: w511 -> [w538 _]
              tunnel: w527 -> [w537 _]
              tunnel: w526 -> [w536 _]
              frame False {
                n171 = case shown="참" w538 {
                  tunnel: w542 -> [w543 w579]
                  tunnel: [w543 w553] -> w541
                  tunnel: w540 -> [_ w569]
                  tunnel: w537 -> [_ w552]
                  tunnel: w536 -> [_ w561]
                  tunnel: w539 -> [_ w546]
                  frame False {
                  }
                  frame True {
                    w555 = 9 items=["xlInsideHorizontal"=12, "xlInsideVertical"=11, "xlDiagonalDown"=5, "xlDiagonalUp"=6, "xlEdgeBottom"=9, "xlEdgeLeft"=7, "xlEdgeRight"=10, "xlEdgeTop"=8] ("Index")
                    n172 = Array Size(array=w546) -> (size(s)=w563:i32[])
                    n173 = Index Array(array=w563) -> (element #1=w562:i32, element #2=w560:i32)  [unwired: 2 in]
                    n174 = Decrement(x=w562) -> (x-1=w559:i32)
                    n175 = Increment(x=w552) -> (x+1=w548:i32)
                    n176 = Add(x=w561, y=w559) -> (x+y=w564:i32)
                    n177 = Add(x=w552, y=w560) -> (x+y=w545:i32)
                    n178 = Bundle(w561, "Column"=w552) -> (w566:cluster{i32, "Column":i32})  [unwired: 1 in]
                    n179 = Decrement(x=w545) -> (x-1=w544:i32)
                    n180 = Bundle(w564, w544) -> (w565:cluster{i32, i32})  [unwired: 1 in]
                    n181 = call <vilib>:"Excel_Get_Range.vi"("Excel._Worksheet"=w569, "start"=w566, "end"=w565, "error in (no error)"=w579) -> ("Range"=w570:refnum<k7>, "error out"=w571:errorcluster)  [unwired: 10 in]
                    n182 = invoke class="Range" method="Value"(reference=w570, error in=w571, "newValue"=w546) -> (reference out=w574:refnum<k7>, error out=w575:errorcluster)  [unwired: 2 in, 3 out]
                    n183 = Less?(x=w544, y=w548) -> (x < y?=w549:bool)
                    n184 = property class="Range"(reference=w574, error in=w575) -> (error out=w577:errorcluster, "Font"=w576:refnum<k7>)  [unwired: 1 out]
                    n185 = Select(t=w548, s=w549, f=w544) -> (s? t:f=w547:i32)
                    n186 = property class="Font"(reference=w576, error in=w577, "Bold"=TRUE) -> (error out=w554:errorcluster)  [unwired: 1 out]
                    n187 = Bundle(w564, w548) -> (w568:cluster{i32, i32})  [unwired: 1 in]
                    n188 = Bundle(w564, w547) -> (w567:cluster{i32, i32})  [unwired: 1 in]
                    n189 = call <vilib>:"Excel_Get_Range.vi"("Excel._Worksheet"=w569, "start"=w568, "end"=w567, "error in (no error)"=w554) -> ("Range"=w573:refnum<k7>, "error out"=w572:errorcluster)  [unwired: 10 in]
                    n190 = property class="Range"(reference=w573, error in=w572) -> (error out=w551:errorcluster, "Borders"=w550:refnum<k7>)  [unwired: 1 out]
                    n191 = invoke class="Borders" method="Item"(reference=w550, error in=w551, "Index"=w555) -> (error out=w558:errorcluster, "Item"=w556:refnum<k7>)  [unwired: 1 in, 2 out]
                    n192 = property class="Border"(reference=w556, error in=w558, "LineStyle"=1) -> (error out=w553:errorcluster)  [unwired: 1 out]
                  }
                }
              }
              frame True {
              }
            }
            n193 = call <vilib>:"Excel_Get_Range.vi"("Excel._Worksheet"=w528, "name"=w512, "error in (no error)"=w529) -> ("Range"=w521:refnum<k7>, "error out"=w522:errorcluster)  [unwired: 11 in]
            n194 = property(reference=w521, error in=w522) -> (error out=w523:errorcluster, "Rows"=w520:refnum<k7>, "Row"=w524:i32)  [unwired: 1 out]
            n195 = Add(x=w526, y=43) -> (x+y=w517:i32)
            n196 = property(reference=w520, error in=w523) -> (error out=w519:errorcluster, "Count"=w525:i32)  [unwired: 1 out]
            n197 = Decrement(x=w525) -> (x-1=w510:i32)
            n198 = Add(x=w510, y=w524) -> (x+y=w518:i32)
            n199 = Less?(x=w518, y=w517) -> (x < y?=w516:bool)
            n200 = Select(t=Cmd_Excel_Insert_Header."Header 넘버링", s=w516, f=Cmd_Excel_Insert_Header."행 삽입") -> (s? t:f=w533:T1)
          }
          frame "Header 넘버링" {
            w584 = 5
            n201 = call <vilib>:"Excel Get Last Row.vi"("report in"=w599, "error in (no error)"=w600) -> ("report out"=w585:refnum<class "NI_report.lvclass">, "MS Office parameters out"=w601:T2, "error out"=w598:errorcluster)  [unwired: 11 in]
            n202 = Unbundle By Name(w601) -> ("position (excel).row"=w602:i32)
            n203 = Greater Or Equal To 0?(x=w587) -> (x >= 0?=w595:bool)
            n204 = Decrement(x=w602) -> (x-1=w583:i32)
            n205 = Select(t=w587, s=w595, f=0) -> (s? t:f=w594:i32)
            n206 = Greater Or Equal?(x=w584, y=w583) -> (x >= y?=w582:bool)
            n207 = case shown="거짓" w582 {
              tunnel: w583 -> [w608 _]
              tunnel: w584 -> [w607 _]
              tunnel: w598 -> [w606 w662]
              tunnel: w596 -> [w605 _]
              tunnel: w594 -> [w604 _]
              tunnel: [w603 w662] -> w586
              frame False {
                n208 = Bundle(w608, "f"=w604) -> (w624:cluster{i32, "f":i32})  [unwired: 1 in]
                n209 = Bundle(w607, "f"=w604) -> (w620:cluster{i32, "f":i32})  [unwired: 1 in]
                n210 = call <vilib>:"Excel_Get_Range.vi"("Excel._Worksheet"=w605, "start"=w620, "end"=w624, "error in (no error)"=w606) -> ("Range"=w610:refnum<k7>, "error out"=w609:errorcluster)  [unwired: 10 in]
                n211 = property class="Range"(reference=w610, error in=w609) -> (reference out=w612:refnum<k7>, error out=w611:errorcluster, "Value2"=w615:variant)
                n212 = Close Reference(reference=w612, error in (no error)=w611) -> (error out=w613:errorcluster)
                n213 = Variant To Data(error in=w613, type=string[][] [], Variant=w615) -> (data=w616:string[][], error out=w618:errorcluster)
                n214 = for {
                  tunnel: w616 -> [w631] mode=indexing
                  shift-right: [w633] -> _
                  shift-left: 0 -> [w628]
                  tunnel: [w629] -> w623 mode=indexing
                  shift-right: [w627] -> w619
                  shift-left: w618 -> [w627]
                  n215 = Index Array(array=w631, index=0 ("인덱스")) -> (element=w634:string)
                  n216 = call <vilib>:"Trim Whitespace.vi"("string"=w634) -> ("trimmed string"=w636:string)  [unwired: 1 in]
                  n217 = Empty String/Path?(string/path=w636) -> (empty?=w635:bool)
                  n218 = case shown="거짓" w635 {
                    tunnel: w634 -> [w645 w660]
                    tunnel: w628 -> [w640 w661]
                    tunnel: [w639 w661] -> w633
                    tunnel: [w646 w660] -> w632
                    frame False {
                      n219 = Search and Replace String(input string=w645, search string="■" ("검색 문자열")) -> (result string=w644:string, offset past replacement=w642:i32)  [unwired: 6 in, 2 out]
                      n220 = Less Than 0?(x=w642) -> (x < 0?=w641:bool)
                      n221 = case shown="거짓" w641 {
                        tunnel: [w653 w659] -> w646
                        tunnel: w644 -> [w650 w659]
                        tunnel: w640 -> [w649 w658]
                        tunnel: [w648 w658] -> w639
                        tunnel: "(Continue)" ("검색 문자열") -> [w647 _]
                        frame False {
                          n222 = Search and Replace String(input string=w650, search string=w647) -> (offset past replacement=w652:i32)  [unwired: 6 in, 3 out]
                          n223 = Less Than 0?(x=w652) -> (x < 0?=w651:bool)
                          n224 = case shown="참" w651 {
                            tunnel: [w655 w657] -> w648
                            tunnel: w649 -> [w655 w656]
                            frame False {
                            }
                            frame True {
                              n225 = Increment(x=w656) -> (x+1=w657:i32)
                            }
                          }
                          n226 = Format Into String(format string="%#f. %s" ("문자열"), w648, w650) -> (resulting string=w653:string)  [unwired: 2 in, 1 out]
                        }
                        frame True {
                        }
                      }
                    }
                    frame True {
                    }
                  }
                  n227 = Replace Array Subset(array=w631, new element=w632, index=0 ("인덱스")) -> (w629:string[])
                }
                n228 = call <vilib>:"Excel_Get_Range.vi"("Excel._Worksheet"=w605, "start"=w620, "end"=w624, "error in (no error)"=w619) -> ("Range"=w622:refnum<k7>, "error out"=w621:errorcluster)  [unwired: 10 in]
                n229 = invoke class="Range" method="Value"(reference=w622, error in=w621, "newValue"=w623) -> (reference out=w626:refnum<k7>, error out=w625:errorcluster)  [unwired: 2 in, 3 out]
                n230 = Close Reference(reference=w626, error in (no error)=w625) -> (error out=w603:errorcluster)
              }
              frame True {
              }
            }
          }
          frame "B_Tag 삽입" {
            n231 = call <vilib>:"Excel_Get_Range.vi"("Excel._Worksheet"=w691, "name"=w699, "error in (no error)"=w707) -> ("Range"=w709:refnum<k7>, "error out"=w708:errorcluster)  [unwired: 11 in]
            n232 = property class="Range"(reference=w709, error in=w708) -> (reference out=w711:refnum<k7>, error out=w710:errorcluster, "Interior"=w685:refnum<k7>, "Columns"=w686:refnum<k7>, "Row"=w679:i32, "Column"=w692:i32)
            n233 = Close Reference(reference=w711, error in (no error)=w710) -> (error out=w682:errorcluster)
            n234 = Decrement(x=w692) -> (x-1=w694:i32)
            n235 = property class="Interior"(reference=w685, error in=w682, "Color"=-4142) -> (reference out=w688:refnum<k7>, error out=w681:errorcluster)
            n236 = Close Reference(reference=w688, error in (no error)=w681) -> (error out=w680:errorcluster)
            n237 = global read "Global_Cal Info.vi" "교정정보"() -> (w666:T3)
            n238 = property class="Range"(reference=w686, error in=w680) -> (reference out=w695:refnum<k7>, error out=w696:errorcluster, "Count"=w698:i32)
            n239 = Subtract(x=w679, y=2) -> (x-y=w684:i32)
            n240 = Unbundle By Name(w666) -> ("영문성적서?"=w665:bool)
            n241 = Decrement(x=w698) -> (x-1=w687:i32)
            n242 = Add(x=w687, y=w694) -> (x+y=w690:i32)
            n243 = Close Reference(reference=w695, error in (no error)=w696) -> (error out=w693:errorcluster)
            n244 = Select(t="End.", s=w665, f="场.") -> (s? t:f=w667:string)
            n245 = Bundle(w684, w690) -> (w697:cluster{i32, i32})  [unwired: 1 in]
            n246 = call <vilib>:"Excel_Get_Range.vi"("Excel._Worksheet"=w691, "start"=w697, "error in (no error)"=w693) -> ("Range"=w713:refnum<k7>, "error out"=w712:errorcluster)  [unwired: 11 in]
            n247 = invoke class="Range" method="Value"(reference=w713, error in=w712, "newValue"=w667) -> (reference out=w678:refnum<k7>, error out=w677:errorcluster)  [unwired: 2 in, 3 out]
            n248 = property class="Range"(reference=w678, error in=w677) -> (reference out=w670:refnum<k7>, error out=w676:errorcluster, "Font"=w675:refnum<k7>)
            n249 = property class="Font"(reference=w675, error in=w676, "Bold"=TRUE) -> (reference out=w671:refnum<k7>, error out=w673:errorcluster)
            n250 = Close Reference(reference=w671, error in (no error)=w673) -> (error out=w672:errorcluster)
            n251 = Close Reference(reference=w670, error in (no error)=w672) -> (error out=w704:errorcluster)
          }
          frame "오류 검사" {
            w739 = T4 0 items=["대화 상자 없음", "확인 메시지", "메시지 지속 또는 정지", "확인 메시지 + 경고", "지속/정지 + 경고"] ("type of dialog (OK msg:1)")
            n252 = call <vilib>:"Excel Get Last Row.vi"("report in"=w725, "error in (no error)"=w727) -> ("report out"=w730:refnum<class "NI_report.lvclass">, "MS Office parameters out"=w728:T2, "error out"=w729:errorcluster)  [unwired: 11 in]
            n253 = Unbundle By Name(w728) -> ("position (excel).row"=w734:i32)
            n254 = Bundle(5, 0) -> (w733:cluster{i32, i32})  [unwired: 1 in]
            n255 = Bundle("row"=w734, 15) -> (w736:cluster{"row":i32, i32})  [unwired: 1 in]
            n256 = call-poly <vilib>:"Excel Get Data.vi"("report in"=w730, "data type"=string[][] [], "start (-1, -1)"=w733, "end (-1, -1)"=w736, "error in (no error)"=w729) -> ("report out"=w716:refnum<class "NI_report.lvclass">, "error out"=w737:errorcluster)  [unwired: 8 in, 1 out]
            n257 = call <vilib>:"Simple Error Handler.vi"("type of dialog (OK msg:1)"=w739, "error in (no error)"=w737) -> ("code out"=w740:i32, "error out"=w741:errorcluster)  [unwired: 3 in, 3 out]
            n258 = case shown="-41117" w740 {
              tunnel: w741 -> [w742 w747]
              tunnel: [w742 w746] -> w726
              tunnel: w715 -> [_ w745]
              frame Default {
              }
              frame -41117 {
                n259 = Format Into String(format string="%s에 오류가 있습니다." ("메시지"), w745) -> (resulting string=w743:string)  [unwired: 2 in, 1 out]
                n260 = call <vilib>:"Clear Errors.vi"("error in (no error)"=w747) -> ("error out"=w746:errorcluster)  [unwired: 5 in, 1 out]
                n261 = One Button Dialog(message=w743) -> ()  [unwired: 1 in, 1 out]
              }
            }
          }
          frame "종료" {
          }
          frame "Error" {
            n262 = Format Into String(w761) -> (resulting string=w762:string)  [unwired: 3 in, 1 out]
            n263 = xnode "에러 링"("파라미터 0"=w762) -> ("에러 출력"=w763:errorcluster)
            n264 = call <vilib>:"Simple Error Handler.vi"("error in (no error)"=w763) -> ("error out"=w765:errorcluster)  [unwired: 4 in, 4 out]
            n265 = call <vilib>:"Clear Errors.vi"("error in (no error)"=w765) -> ("error out"=w764:errorcluster)  [unwired: 5 in, 1 out]
          }
        }
        n266 = Unbundle By Name(w20) -> ("status"=w23:bool)
        n267 = Greater?(x=w42, y=100) -> (0:w40:bool)
        n268 = call "stop.vi"("cmd (read)"=enum16{"write", "read"}."write", "error in (no error)"=w20, "stop"=w40) -> ("error out"=w35:errorcluster, "stop?"=w43:bool)  [unwired: 7 in]
        n269 = Select(t=Cmd_Excel_Insert_Header."Error" ("f"), s=w23, f=w18) -> (s? t:f=w22:T1)
        n270 = Compound Arithmetic op=OR(w43, w44) -> (w45:bool)
        "?" <- w30
      }
    }
    frame Error {
    }
  }
  "error out" <- w2
  "report out" <- w3
